vi "HAR-15-001-RecordingStimulation_BL.vi"() -> ()   [LabVIEW 2014]
doc: "I. Description:\nThis example demonstrates how to continuously acquire unscaled and save the data in a binary file. You can use the Graph Acquired Binary Data.VI to read and plot the scaled data on a Waveform Graph.\n\nII. Instructions for Running:\n1. Select the physical channel to correspond to where your signal is input on the DAQ device.\n2. Enter the minimum and maximum voltage ranges.\nNote: For better accuracy try to match the input range to the expected voltage level of the measured signal.\n3. Set the rate of the acquisition Also set the Samples to Read control. This will determine how many samples are read each time the while loop iterates. This also determines how many points are plotted on the graph each iteration.\nNote: The rate should be at least twice as fast as the maximum frequency component of the signal being acquired.\n4. Select the File Properties. If the file path is left empty, it will bring up a dialog box to let you browse to the file. \n\nIII. Block Diagram Steps:\n1. Create or replace a file to store the data.\n2. Create an analog input voltage channel.\n3. Set the rate for the sample clock. Additionally, define the sample mode to be continuous.\n4. Create a header and write it to the binary file.\n5. Call the Start VI to start acquiring samples. \n6. Read the unscaled data in a loop until the user hits the stop button or an error occurs.\nNote: This example uses unscaled I32 reads. Some devices support unscaled reads in smaller widths, such as I16. To get the maximum performance out of your device, use the unscaled read with the smallest supported width.\n7. Transpose the unscaled array of data and append it to the file.\n8. Close the File.\n9. Call the Stop VI to stop acquiring samples.\n10. Use the popup dialog box to display an error if any.\n\nIV. I/O Connections Overview:\nMake sure your signal input terminal matches the Physical Channel I/O control. For further connection information, refer to your hardware reference manual."
uses:
  <vilib>/Utility/error.llb/DialogType.ctl
  <vilib>/DAQmx/read.llb/DAQmx Read (Analog 2D I32 NChan NSamp).vi
  <vilib>/DAQmx/create/channels.llb/DAQmx Create Channel (AI-Voltage-Basic).vi
  <vilib>/DAQmx/configure/timing.llb/DAQmx Timing (Sample Clock).vi
  <vilib>/DAQmx/miscellaneous.llb/DAQmx Fill In Error Info.vi
  <vilib>/Utility/file.llb/Read From Spreadsheet File (string).vi
  <vilib>/Waveform/DWDTOps.llb/DWDT Boolean Array to Digital.vi
panel:
  out "AMP Thres":dbl
  in  "WinEnd":i32
  in  "WinStart":i32
  in  "Y Scale Range":dbl=10.0
  out "StimulationCounter":i32
  out "?":i32
  in  "?":u16(ring) items=["TC1", "TC2", "TC3", "TC4", "TC5", "TC6", "TC7", "TC8", "TC9", "TC10"]
  out "TC On?":bool
  in  "?":bool
  out "Orders":i32[][](array[numeric])
  out "StimulationSetting":T1(array[cluster])
  in  "?":enum32{"ES1", "ES 2", "TMS"}(radio)
  out "Files Opens":bool[](array[boolean])
  out "1st Event Position":dbl
  out "Group of ES set":i32
  out "File Writing Array":bool[](array[boolean])
  out "Single File RefNum":refnum<file>
  out "Files RefNum":refnum<file>[](array[refnum])
  out "Cursor Auto Jump":bool
  in  "Curor Auto Jump":bool=TRUE
  in  "?":bool
  out "STDP On?":bool
  out "# Events":u32
  out "# Reps Left":dbl
  in  "Tab Control":T2(tab)
  out "R APB":dbl[][](graph)
  out "R ADM":dbl[][](graph)
  out "R APB AMP":dbl
  out "R ADM AMP":dbl
  out "R APB +":i32
  out "R APB -":i32
  out "R ADM -":i32
  out "R ADM +":i32
  out "L ADM -":i32
  out "L ADM +":i32
  out "L APB -":i32
  out "L APB +":i32
  out "L ADM AMP":dbl
  out "L APB AMP":dbl
  out "L APB":dbl[][](graph)
  out "L ADM":dbl[][](graph)
  out "R BI":dbl[][](graph)
  out "R BI AMP":dbl
  out "R BI +":i32
  out "R BI -":i32
  out "L BI":dbl[][](graph)
  out "L BI -":i32
  out "L BI +":i32
  out "L BI AMP":dbl
  out "L FCR":dbl[][](graph)
  out "L FCR AMP":dbl
  out "L FCR +":i32
  out "L FCR -":i32
  out "R FCR":dbl[][](graph)
  out "R FCR -":i32
  out "R FCR +":i32
  out "R FCR AMP":dbl
  out "Looping Iteration":i16
  in  "Repetitions":i8=5
  in  "TMS Delay Interval":dbl max=250.0
  out "TMS Delay Interval (ms)":dbl(slide) scale=0.0..250.0
  in  "TMS Interval":dbl=40.0
  out "ES 2 Delay Interval (ms)":dbl(slide) scale=0.0..250.0
  in  "ES2 Delay Interval":dbl max=250.0
  in  "ES2 Interval":dbl=40.0
  in  "ES1 Delay Interval":dbl max=250.0
  out "ES 1 Delay Interval (ms)":dbl(slide) max=100.0 scale=0.0..250.0
  in  "ES1 Interval":dbl=40.0
  in  "Trigger Pulse Width (Points)":i16=5
  in  "Rate - every X s":dbl=5.0
  in  "?":bool
  in  "Looping Switch":bool
  in  "Buffered Size":i16=2500
  in  "Sampling Rate":dbl=10000.0
  out "ES1 On?":bool
  out "ES2 On?":bool
  out "TMS On?":bool
  in  "TMS Activate":bool=TRUE
  in  "ES1 Activate":bool=TRUE
  in  "ES2 Activate":bool=TRUE
  out "ES1 DP On?":bool
  out "ES2 DP On?":bool
  out "TMS Doublet On?":bool
  in  "ES1 Doublet On?":bool
  in  "ES2 Doublet On?":bool
  in  "TMS Doublet On?":bool
  out "peak X value":dbl
  out "Peak Count":i32
  in  "peak number":i32
  in  "Cursor Jump":bool
  out "S1":dbl[][](graph)
  in  "stop B":bool
  in  "stop A":bool
  in  "# updates/sec":dbl=4.0
  out "volts/bit":dbl
  out "Samples Per Channel Per Iteration":dbl
  out "Time (sec)":dbl
  out "# channels":dbl
  out "Samples to Read":i32=1
  in  "Maximum Value":dbl=10.0 format="%0.2f"
  in  "Minimum Value":dbl=-10.0 format="%0.2f"
  in  "DAQ Channels":tag="Dev3/ai0:7, Dev3/ai16:18" caption="Channel List"
  # "File Properties"
  # "Channel Parameters"
  # "Advanced Setting For DO"
  # "Timing Parameters"
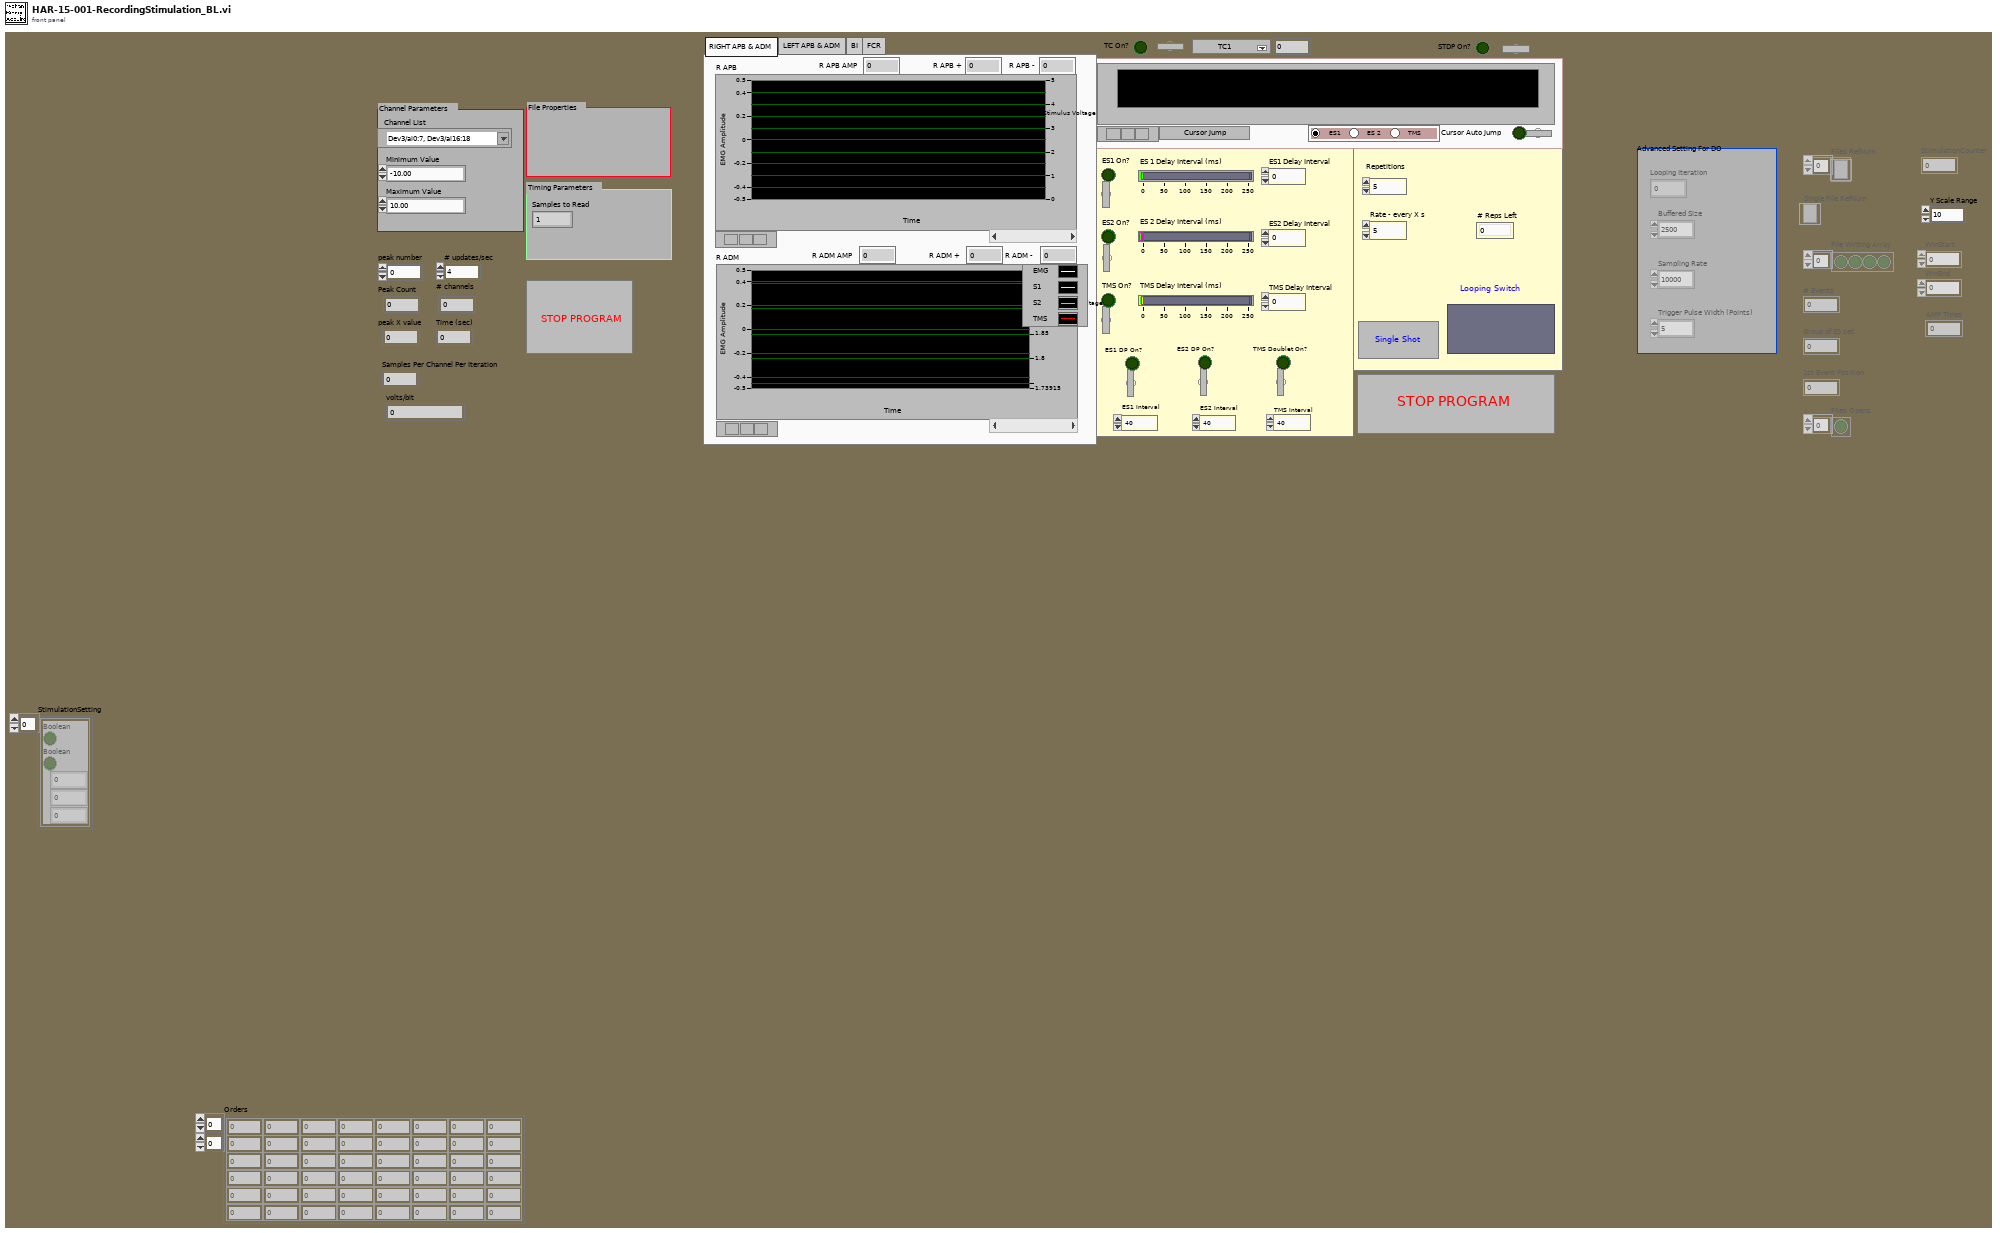
[diagram p1: front panel]
types:
  T1 = cluster{"Boolean":bool, "Boolean":bool, dbl, dbl, dbl}[]
  T2 = enum32{"RIGHT APB & ADM", "LEFT APB & ADM", "BI", "FCR"}
  T3 = typedef "DialogType.ctl" = u16
  T4 = cluster{"Boolean":bool, "Boolean":bool, dbl, dbl, dbl}
  T5 = enum16{"open", "open or create", "create or replace", "create", "open (read only)"}
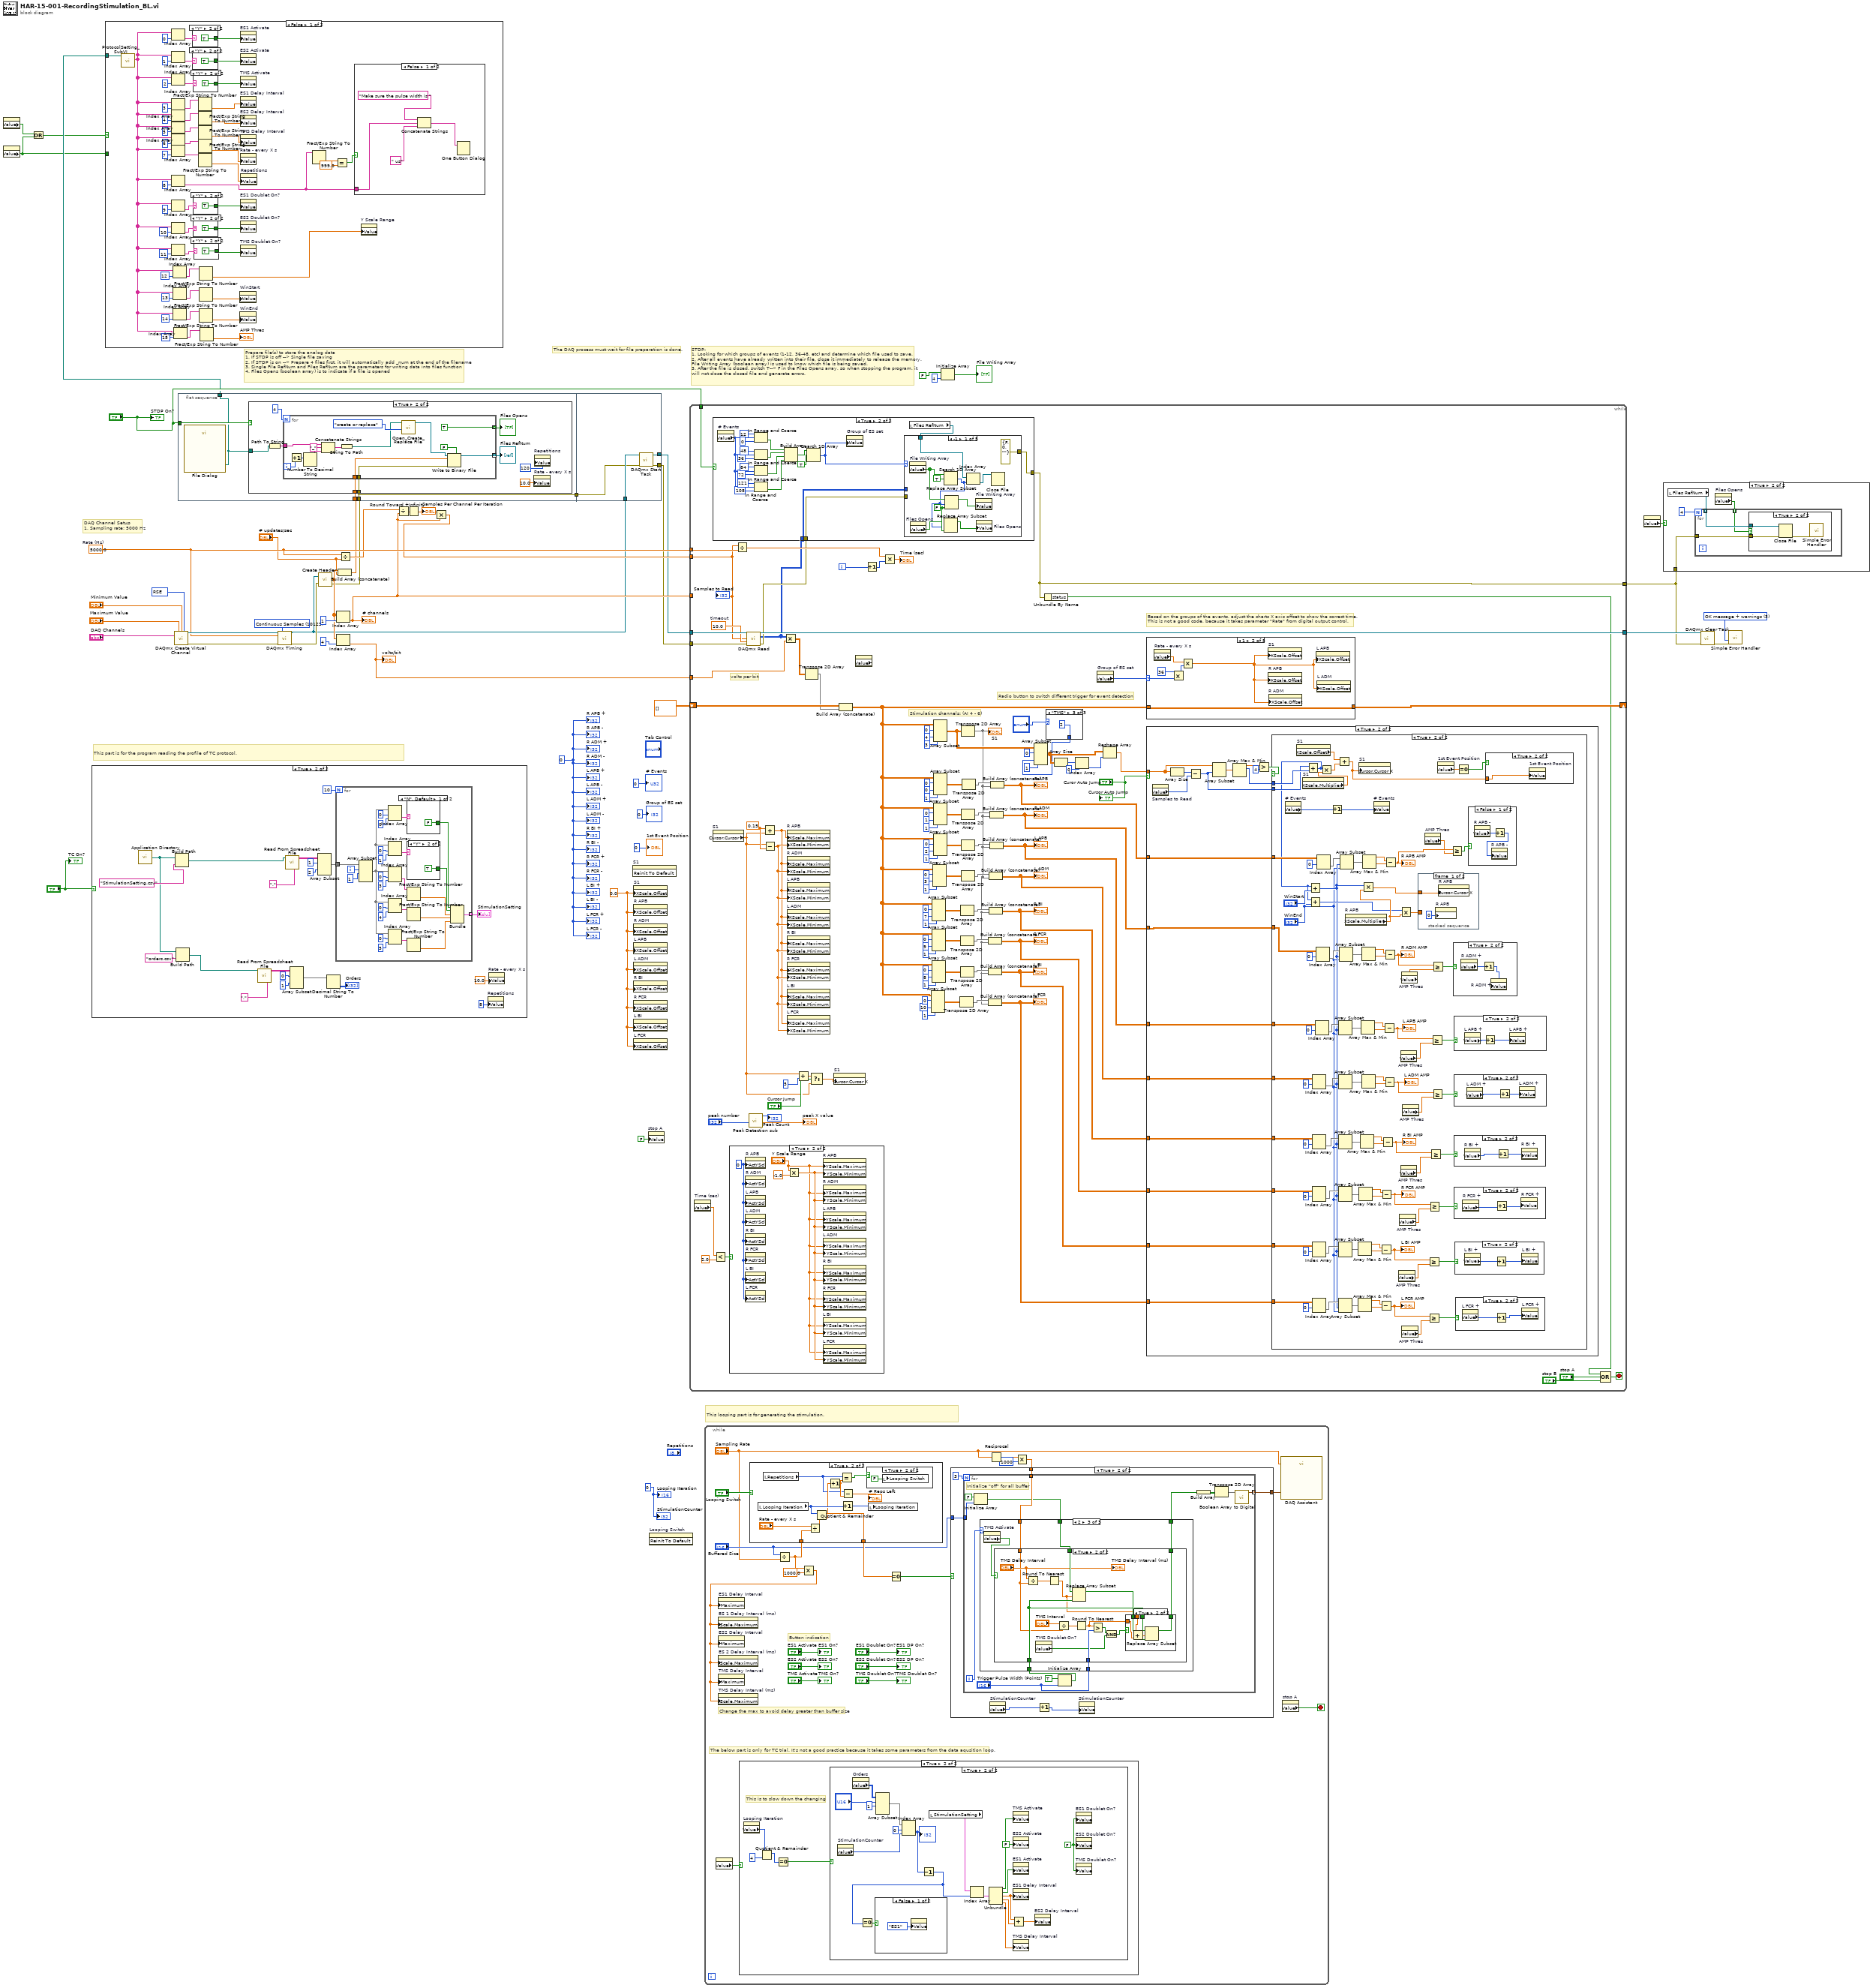
[diagram p0: block diagram]
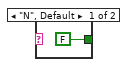
[diagram p3: hidden frame]
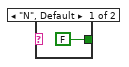
[diagram p4: hidden frame]
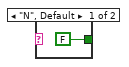
[diagram p5: hidden frame]
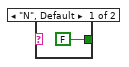
[diagram p6: hidden frame]
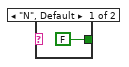
[diagram p7: hidden frame]
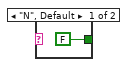
[diagram p8: hidden frame]
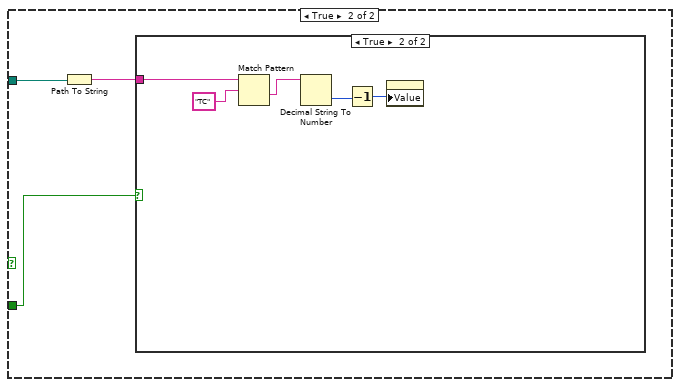
[diagram p9: hidden frame]
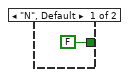
[diagram p12: hidden frame]
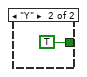
[diagram p13: hidden frame]
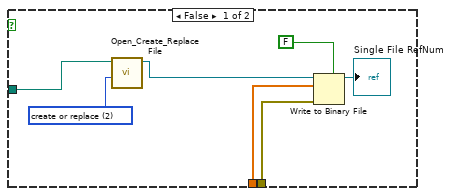
[diagram p14: hidden frame]
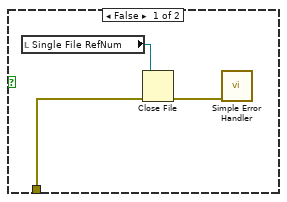
[diagram p15: hidden frame]
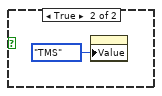
[diagram p19: hidden frame]
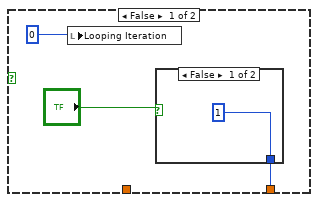
[diagram p20: hidden frame]
diagram:
  w2 = 0
  w1 = 0.0 ("X Scale.Offset and Multiplier:Offset")
  w10 = 0
  w35 = 5000.0  # Rate (Hz)
  w41 = 10083 items=["default"=-1, "RSE"=10083, "NRSE"=10078, "Differential"=10106, "Pseudodifferential"=12529] ("input terminal configuration")
  w43 = T3 3 items=["no dialog", "OK message", "continue or stop message", "OK message + warnings", "continue/stop + warnings"] ("type of dialog (OK msg:1)")
  w45 = 10123 items=["Finite Samples"=10178, "Continuous Samples"=10123] ("sample mode")
  # "This looping part is for generating the stimulation."
  # "This part is for the program reading the profile of TC protocol."
  # "STDP:\n1. Looking for which groups of events (1-12, 36-48, etc) and determine which file used to save.\n2. After all events have already written into their file, close it immediately to release the memory.\nFile Writing Array (boolean array) is used to know which file is being saved.\n3. After the file is closed, switch T--> F in the Files Opens array, so when stopping the program, it\nwill not close the closed file and generate errors."
  # "The DAQ process must wait for file preparation is done."
  # "DAQ Channel Setup\n1. Sampling rate: 5000 Hz"
  # "Prepare file(s) to store the analog data\n1. If STDP is off --> Single file saving\n2. If STDP is on --> Prepare 4 files first, it will automatically add _num at the end of the filename\n3. Single File RefNum and Files RefNum are the parameters for writing data into files function\n4. Files Opens (boolean array) is to indicate if a file is opened"
  n1 = property class="Bool (strict)"() -> ("Value"=w6:bool)  [unwired: 2 in, 2 out]
  n2 = property class="Bool (strict)"() -> ("Value"=w3:bool)  [unwired: 2 in, 2 out]
  n3 = Or(x=w6, y=w3) -> (x .or. y?=w5:bool)
  n4 = case shown="True" "?" {
    frame False {
    }
    frame True {
      n5 = call <vilib>:"Application Directory.vi"() -> ("Application Directory"=w50:path)
      n6 = Build Path(base path=w50, name or relative path="StimulationSetting.csv" ("file path (dialog if empty)")) -> (appended path=w51:path)
      n7 = Build Path(base path=w50, name or relative path="orders.csv") -> (appended path=w48:path)
      n8 = call-poly <vilib>:"Read From Spreadsheet File.vi"("delimiter (\\t)"="," ("delimiter (\\t)"), "file path (dialog if empty)"=w48) -> ("all rows"=w59:string[][])  [unwired: 5 in, 4 out]
      n9 = call-poly <vilib>:"Read From Spreadsheet File.vi"("delimiter (\\t)"="," ("delimiter (\\t)"), "file path (dialog if empty)"=w51) -> ("all rows"=w66:string[][])  [unwired: 5 in, 4 out]
      n10 = Array Subset(array=w59, index (row)=0 ("index"), index (col)=1 ("index")) -> (w56:string[][])  [unwired: 2 in]
      n11 = Array Subset(array=w66, index (row)=1 ("index"), index (col)=2 ("index")) -> (w63:string[][])  [unwired: 2 in]
      n12 = Decimal String To Number(string=w56) -> (number=→"Orders":i32[][])  [unwired: 2 in, 1 out]
      n13 = for {
        N: 10 -> [_]
        tunnel: w63 -> [w92]
        tunnel: [w68] -> w61 mode=indexing
        i -> [w74]
        n14 = Array Subset(array=w92, index (row)=w74, length (row)=1 ("length")) -> (w78:string[][])  [unwired: 2 in]
        n15 = Index Array(array=w78, index (row)=0, index (col)=0 ("disabled index (col)")) -> (element=w88:string)
        n16 = Index Array(array=w78, index (row)=0, index (col)=1 ("disabled index (col)")) -> (element=w85:string)
        n17 = Index Array(array=w78, index (row)=0, index (col)=3 ("disabled index (col)")) -> (element=w75:string)
        n18 = Index Array(array=w78, index (row)=0, index (col)=4 ("disabled index (col)")) -> (element=w76:string)
        n19 = Index Array(array=w78, index (row)=0, index (col)=5 ("disabled index (col)")) -> (element=w77:string)
        n20 = case shown="\"N\", Default" w88 {
          tunnel: [FALSE ("Boolean") TRUE ("Boolean")] -> w73
          frame "N", Default {
          }
          frame "Y" {
          }
        }
        n21 = case shown="\"Y\"" w85 {
          tunnel: [FALSE ("Boolean") TRUE ("Boolean")] -> w72
          frame "N", Default {
          }
          frame "Y" {
          }
        }
        n22 = Fract/Exp String To Number(string=w75) -> (number=w71:dbl)  [unwired: 3 in, 1 out]
        n23 = Fract/Exp String To Number(string=w76) -> (number=w70:dbl)  [unwired: 3 in, 1 out]
        n24 = Fract/Exp String To Number(string=w77) -> (number=w69:dbl)  [unwired: 3 in, 1 out]
        n25 = Bundle("Boolean"=w73, "Boolean"=w72, w71, w70, w69) -> (w68:T4)  [unwired: 1 in]
      }
      "StimulationSetting" <- w61
      n26 = property on="Repetitions" class="DigNum (strict)"("Value"=i8 8 ("Repetitions")) -> ()  [unwired: 2 in, 2 out]
      n27 = property on="Rate - every X s" class="DigNum (strict)"("Value"=10.0 ("Rate - every X s")) -> ()  [unwired: 2 in, 2 out]
    }
  }
  n28 = case shown="False" w5 {
    tunnel: w9 -> [w117 w166]
    tunnel: w3 -> [_ w165]
    frame False {
      n29 = call "ProtocolSetting_SubVI.vi"("selected path"=w117) -> ("all rows"=w99:string[])  [unwired: 9 in, 1 out]
      n30 = Index Array(array=w99, index=0) -> (element=w147:string)
      n31 = Index Array(array=w99, index=1) -> (element=w144:string)
      n32 = Index Array(array=w99, index=2) -> (element=w142:string)
      n33 = Index Array(array=w99, index=3) -> (element=w139:string)
      n34 = Index Array(array=w99, index=4) -> (element=w138:string)
      n35 = Index Array(array=w99, index=5) -> (element=w137:string)
      n36 = Index Array(array=w99, index=6) -> (element=w136:string)
      n37 = Index Array(array=w99, index=7) -> (element=w132:string)
      n38 = Index Array(array=w99, index=8) -> (element=w110:string)
      n39 = Index Array(array=w99, index=9) -> (element=w131:string)
      n40 = Index Array(array=w99, index=10) -> (element=w130:string)
      n41 = Index Array(array=w99, index=11) -> (element=w129:string)
      n42 = Index Array(array=w99, index=12) -> (element=w108:string)
      n43 = Index Array(array=w99, index=13) -> (element=w104:string)
      n44 = Index Array(array=w99, index=14) -> (element=w103:string)
      n45 = Index Array(array=w99, index=15) -> (element=w98:string)
      n46 = case shown="\"Y\"" w147 {
        tunnel: [FALSE TRUE] -> w146
        frame "N", Default {
        }
        frame "Y" {
        }
      }
      n47 = case shown="\"Y\"" w144 {
        tunnel: [FALSE TRUE] -> w141
        frame "N", Default {
        }
        frame "Y" {
        }
      }
      n48 = case shown="\"Y\"" w142 {
        tunnel: [FALSE TRUE] -> w140
        frame "N", Default {
        }
        frame "Y" {
        }
      }
      n49 = case shown="\"Y\"" w131 {
        tunnel: [FALSE TRUE] -> w120
        frame "N", Default {
        }
        frame "Y" {
        }
      }
      n50 = case shown="\"Y\"" w130 {
        tunnel: [FALSE TRUE] -> w119
        frame "N", Default {
        }
        frame "Y" {
        }
      }
      n51 = case shown="\"Y\"" w129 {
        tunnel: [FALSE TRUE] -> w118
        frame "N", Default {
        }
        frame "Y" {
        }
      }
      n52 = Fract/Exp String To Number(string=w139) -> (number=w135:dbl)  [unwired: 3 in, 1 out]
      n53 = Fract/Exp String To Number(string=w138) -> (number=w134:dbl)  [unwired: 3 in, 1 out]
      n54 = Fract/Exp String To Number(string=w137) -> (number=w133:dbl)  [unwired: 3 in, 1 out]
      n55 = Fract/Exp String To Number(string=w136) -> (number=w115:dbl)  [unwired: 3 in, 1 out]
      n56 = Fract/Exp String To Number(string=w132) -> (number=w114:dbl)  [unwired: 3 in, 1 out]
      n57 = Fract/Exp String To Number(string=w108) -> (number=w107:dbl)  [unwired: 3 in, 1 out]
      n58 = Fract/Exp String To Number(string=w104) -> (number=w102:dbl)  [unwired: 3 in, 1 out]
      n59 = Fract/Exp String To Number(string=w103) -> (number=w101:dbl)  [unwired: 3 in, 1 out]
      n60 = Fract/Exp String To Number(string=w98) -> (number=→"AMP Thres":dbl)  [unwired: 3 in, 1 out]
      n61 = property on="WinStart" class="DigNum (strict)"("Value"=w102) -> ()  [unwired: 2 in, 2 out]
      n62 = property on="WinEnd" class="DigNum (strict)"("Value"=w101) -> ()  [unwired: 2 in, 2 out]
      n63 = property on="ES1 Activate" class="Bool (strict)"("Value"=w146) -> ()  [unwired: 2 in, 2 out]
      n64 = property on="ES2 Activate" class="Bool (strict)"("Value"=w141) -> ()  [unwired: 2 in, 2 out]
      n65 = property on="TMS Activate" class="Bool (strict)"("Value"=w140) -> ()  [unwired: 2 in, 2 out]
      n66 = property on="ES1 Delay Interval" class="DigNum (strict)"("Value"=w135) -> ()  [unwired: 2 in, 2 out]
      n67 = property on="ES2 Delay Interval" class="DigNum (strict)"("Value"=w134) -> ()  [unwired: 2 in, 2 out]
      n68 = property on="TMS Delay Interval" class="DigNum (strict)"("Value"=w133) -> ()  [unwired: 2 in, 2 out]
      n69 = property on="Rate - every X s" class="DigNum (strict)"("Value"=w115) -> ()  [unwired: 2 in, 2 out]
      n70 = property on="ES1 Doublet On?" class="Bool (strict)"("Value"=w120) -> ()  [unwired: 2 in, 2 out]
      n71 = property on="ES2 Doublet On?" class="Bool (strict)"("Value"=w119) -> ()  [unwired: 2 in, 2 out]
      n72 = property on="TMS Doublet On?" class="Bool (strict)"("Value"=w118) -> ()  [unwired: 2 in, 2 out]
      n73 = property on="Repetitions" class="DigNum (strict)"("Value"=w114) -> ()  [unwired: 2 in, 2 out]
      n74 = Fract/Exp String To Number(string=w110) -> (number=w113:dbl)  [unwired: 3 in, 1 out]
      n75 = Equal?(x=w113, y=999.0) -> (x = y?=w111:bool)
      n76 = case shown="False" w111 {
        tunnel: w110 -> [w152 _]
        frame False {
          n77 = Concatenate Strings("Make sure the pulse width is ", w152, " us" ("string")) -> (w149:string)
          n78 = One Button Dialog(message=w149) -> ()  [unwired: 1 in, 1 out]
        }
        frame True {
        }
      }
      n79 = property on="Y Scale Range" class="DigNum (strict)"("Value"=w107) -> ()  [unwired: 2 in, 2 out]
    }
    frame True {
      n80 = Path To String(path=w166) -> (string=w167:string)
      n81 = case shown="True" w165 {
        tunnel: w167 -> [_ w172]
        frame False {
        }
        frame True {
          n82 = Match Pattern(string=w172, regular expression="TC") -> (after substring=w170:string)  [unwired: 1 in, 3 out]
          n83 = Decimal String To Number(string=w170) -> (number=w169:i32)  [unwired: 2 in, 1 out]
          n84 = Decrement(x=w169) -> (x-1=w168:i32)
          n85 = property class="Ring (strict)"("Value"=w168) -> ()  [unwired: 2 in, 2 out]
        }
      }
    }
  }
  n86 = call-poly <vilib>:"DAQmx Create Virtual Channel.vi"("maximum value"="Maximum Value", "minimum value"="Minimum Value", "input terminal configuration"=w41, "physical channels"="DAQ Channels") -> ("task out"=w40:refnum<k21>, "error out"=w39:errorcluster)  [unwired: 5 in, 5 out]
  n87 = flat-sequence {
    tunnel: [w176] -> w8
    tunnel: [w173] -> w9
    tunnel: w21 -> [w176]
    tunnel: w23 -> [w174]
    tunnel: "?" -> [w175]
    tunnel: [w210] -> w20
    tunnel: [w209] -> w19
    tunnel: w7 -> [w208]
    tunnel: w8 -> [w207]
    frame #0 {
      n88 = call "File Dialog"() -> ("selected path"=w173:path)  [unwired: 12 in, 3 out]
      n89 = case shown="True" w175 {
        tunnel: w174 -> [w183 w190]
        tunnel: w176 -> [w180 w189]
        tunnel: w173 -> [w177 w186]
        frame False {
          w179 = i16 2 items=["open", "open or create", "create or replace", "create"] ("function")
          n90 = call <vilib>:"Open_Create_Replace File.vi"("function (open:0)"=w179, "file path"=w177) -> ("refnum"=w178:refnum<file>)  [unwired: 4 in, 5 out]
          n91 = Write to Binary File(file (use dialog)=w178, data=w183, error in=w180, 5:FALSE ("prepend array or string size? (T)")) -> (refnum out=→"Single File RefNum":refnum<file>)  [unwired: 4 out]
        }
        frame True {
          n92 = Path To String(path=w186) -> (string=w192:string)
          n93 = for {
            N: 4 -> [_]
            tunnel: w192 -> [w206]
            tunnel: [w196] -> w188 mode=indexing
            tunnel: w190 -> [w195]
            tunnel: w189 -> [w194]
            tunnel: [TRUE] -> w187 mode=indexing
            i -> [w205]
            n94 = Increment(x=w205) -> (x+1=w204:i32)
            n95 = Number To Decimal String(number=w204) -> (decimal integer string=w203:string)  [unwired: 1 in]
            n96 = Concatenate Strings(w206, "_" ("string"), w203) -> (w200:string)
            n97 = String To Path(string=w200) -> (path=w198:path)
            n98 = call <vilib>:"Open_Create_Replace File.vi"("function (open:0)"=T5."create or replace", "file path"=w198) -> ("refnum"=w197:refnum<file>)  [unwired: 4 in, 5 out]
            n99 = Write to Binary File(file (use dialog)=w197, data=w195, error in=w194, 5:FALSE ("prepend array or string size? (T)")) -> (refnum out=w196:refnum<file>)  [unwired: 4 out]
          }
          "Files RefNum" <- w188
          "Files Opens" <- w187
          n100 = property on="Rate - every X s" class="DigNum (strict)"("Value"=10.0 ("Rate - every X s")) -> ()  [unwired: 2 in, 2 out]
          n101 = property on="Repetitions" class="DigNum (strict)"("Value"=i8 120 ("Repetitions")) -> ()  [unwired: 2 in, 2 out]
        }
      }
    }
    frame #1 {
      n102 = call <vilib>:"DAQmx Start Task.vi"("task/channels in"=w208, "error in"=w207) -> ("task out"=w210:refnum<k21>, "error out"=w209:errorcluster)  [unwired: 12 out]
    }
  }
  n103 = call-poly <vilib>:"DAQmx Timing.vi"("task/channels in"=w40, "sample mode"=w45, "rate"=w35, "error in"=w39) -> ("task out"=w7:refnum<k21>, "error out"=w44:errorcluster)  [unwired: 3 in, 7 out]
  n104 = call "Create Header.vi"("task in"=w7, "error in"=w44) -> ("Array"=w27:dbl[], "error out"=w21:errorcluster)  [unwired: 1 out]
  n105 = Index Array(array=w27, index=1) -> (element=w31:dbl)
  "# channels" <- w31
  n106 = Index Array(array=w27, index=4) -> (element=w28:dbl)
  "volts/bit" <- w28
  n107 = Build Array (concatenate)(w27, "# updates/sec") -> (w23:dbl[])
  n108 = Divide(x=w35, y="# updates/sec") -> (x/y=w34:dbl)
  n109 = Divide(x=w34, y=w31) -> (x/y=w33:dbl)
  n110 = Round Toward +Infinity(x=w33) -> (ceil(x): smallest int >= x=w32:dbl)
  "Samples Per Channel Per Iteration" <- w32
  n111 = Multiply(x=w32, y=w31) -> (x*y=w30:dbl)
  n112 = invoke on="S1" class="WFGraph (strict)" method="Reinit To Default"() -> ()  [unwired: 3 in, 3 out]
  n113 = property on="S1" class="WFGraph (strict)"("XScale.Offset"=w1) -> ()  [unwired: 2 in, 2 out]
  n114 = property on="R APB" class="WFGraph (strict)"("XScale.Offset"=w1) -> ()  [unwired: 2 in, 2 out]
  n115 = property on="R ADM" class="WFGraph (strict)"("XScale.Offset"=w1) -> ()  [unwired: 2 in, 2 out]
  n116 = property on="L APB" class="WFGraph (strict)"("XScale.Offset"=w1) -> ()  [unwired: 2 in, 2 out]
  n117 = property on="L ADM" class="WFGraph (strict)"("XScale.Offset"=w1) -> ()  [unwired: 2 in, 2 out]
  n118 = property on="R BI" class="WFGraph (strict)"("XScale.Offset"=w1) -> ()  [unwired: 2 in, 2 out]
  n119 = property on="R FCR" class="WFGraph (strict)"("XScale.Offset"=w1) -> ()  [unwired: 2 in, 2 out]
  n120 = property on="L BI" class="WFGraph (strict)"("XScale.Offset"=w1) -> ()  [unwired: 2 in, 2 out]
  n121 = property on="L FCR" class="WFGraph (strict)"("XScale.Offset"=w1) -> ()  [unwired: 2 in, 2 out]
  n122 = property on="stop A" class="Bool (strict)"("Value"=FALSE ("stop A")) -> ()  [unwired: 2 in, 2 out]
  n123 = invoke on="Looping Switch" class="Bool (strict)" method="Reinit To Default"() -> ()  [unwired: 3 in, 3 out]
  n124 = while {
    tunnel: w19 -> [w312]
    tunnel: w20 -> [w311]
    tunnel: [w310] -> w47
    tunnel: [w295] -> w13
    tunnel: w31 -> [_]
    tunnel: w28 -> [w297]
    tunnel: w35 -> [w308]
    tunnel: w30 -> [w307]
    tunnel: "?" -> [w299]
    shift-right: [w250] -> _
    shift-left: dbl[][] [] -> [w298]
    i -> [w306]
    stop <- w244 stop-if-true
    w293 = 0.15
    w309 = 10.0  # timeout
    # "Based on the groups of the events, adjust the charts X axis offset to show the correct time.\nThis is not a good code, because it takes parameter \"Rate\" from digital output control."
    # "Radio button to switch different trigger for event detection"
    # "Stimulation channels: (AI 4 - 6)"
    # "volts per bit"
    n125 = property on="Time (sec)" class="DigNum (strict)"() -> ("Value"=w212:dbl)  [unwired: 2 in, 2 out]
    n126 = property on="S1" class="WFGraph (strict)"() -> ("Cursor.Cursor X"=w288:dbl)  [unwired: 2 in, 2 out]
    n127 = Less?(x=w212, y=2.0) -> (x < y?=w213:bool)
    n128 = case shown="True" w213 {
      frame False {
      }
      frame True {
        w315 = 0 ("Active Y Scale")
        n129 = property on="R APB" class="WFGraph (strict)"("ActYScl"=w315) -> ()  [unwired: 2 in, 2 out]
        n130 = property on="R ADM" class="WFGraph (strict)"("ActYScl"=w315) -> ()  [unwired: 2 in, 2 out]
        n131 = property on="L APB" class="WFGraph (strict)"("ActYScl"=w315) -> ()  [unwired: 2 in, 2 out]
        n132 = property on="L ADM" class="WFGraph (strict)"("ActYScl"=w315) -> ()  [unwired: 2 in, 2 out]
        n133 = property on="R BI" class="WFGraph (strict)"("ActYScl"=w315) -> ()  [unwired: 2 in, 2 out]
        n134 = property on="R FCR" class="WFGraph (strict)"("ActYScl"=w315) -> ()  [unwired: 2 in, 2 out]
        n135 = property on="L BI" class="WFGraph (strict)"("ActYScl"=w315) -> ()  [unwired: 2 in, 2 out]
        n136 = property on="L FCR" class="WFGraph (strict)"("ActYScl"=w315) -> ()  [unwired: 2 in, 2 out]
        n137 = Multiply(x="Y Scale Range", y=-1.0) -> (x*y=w314:dbl)
        n138 = property on="R APB" class="WFGraph (strict)"("YScale.Maximum"="Y Scale Range", "YScale.Minimum"=w314) -> ()  [unwired: 2 in, 2 out]
        n139 = property on="R ADM" class="WFGraph (strict)"("YScale.Maximum"="Y Scale Range", "YScale.Minimum"=w314) -> ()  [unwired: 2 in, 2 out]
        n140 = property on="L APB" class="WFGraph (strict)"("YScale.Maximum"="Y Scale Range", "YScale.Minimum"=w314) -> ()  [unwired: 2 in, 2 out]
        n141 = property on="L ADM" class="WFGraph (strict)"("YScale.Maximum"="Y Scale Range", "YScale.Minimum"=w314) -> ()  [unwired: 2 in, 2 out]
        n142 = property on="R BI" class="WFGraph (strict)"("YScale.Maximum"="Y Scale Range", "YScale.Minimum"=w314) -> ()  [unwired: 2 in, 2 out]
        n143 = property on="R FCR" class="WFGraph (strict)"("YScale.Maximum"="Y Scale Range", "YScale.Minimum"=w314) -> ()  [unwired: 2 in, 2 out]
        n144 = property on="L BI" class="WFGraph (strict)"("YScale.Maximum"="Y Scale Range", "YScale.Minimum"=w314) -> ()  [unwired: 2 in, 2 out]
        n145 = property on="L FCR" class="WFGraph (strict)"("YScale.Maximum"="Y Scale Range", "YScale.Minimum"=w314) -> ()  [unwired: 2 in, 2 out]
      }
    }
    n146 = Divide(x=w307, y=w308) -> (x/y=w303:dbl)
    n147 = call-poly <vilib>:"DAQmx Read.vi"("task/channels in"=w311, "number of samples per channel"=w307, "timeout"=w309, "error in"=w312) -> ("task out"=w310:refnum<k21>, "data"=w294:i32[][], "error out"=w300:errorcluster)  [unwired: 9 out]
    n148 = case shown="True" w299 {
      tunnel: w294 -> [w488 w493]
      tunnel: w300 -> [w486 w492]
      tunnel: [w484 w491] -> w295
      frame False {
        n149 = local read "Single File RefNum"() -> (w485:refnum<file>)
        n150 = Write to Binary File(file (use dialog)=w485, data=w488, error in=w486, 5:FALSE ("prepend array or string size? (T)")) -> (error out=w484:errorcluster)  [unwired: 4 out]
      }
      frame True {
        n151 = property on="# Events" class="DigNum (strict)"() -> ("Value"=w500:u32)  [unwired: 2 in, 2 out]
        n152 = In Range and Coerce(upper limit=u32 12, x=w500, lower limit=u32 0) -> (In Range?=w499:bool)  [unwired: 1 out]
        n153 = In Range and Coerce(upper limit=u32 48, x=w500, lower limit=u32 36) -> (In Range?=w498:bool)  [unwired: 1 out]
        n154 = In Range and Coerce(upper limit=u32 84, x=w500, lower limit=u32 72) -> (In Range?=w497:bool)  [unwired: 1 out]
        n155 = In Range and Coerce(upper limit=u32 121, x=w500, lower limit=u32 108) -> (In Range?=w496:bool)  [unwired: 1 out]
        n156 = Build Array(w499, w498, w497, w496) -> (w495:bool[])
        n157 = Search 1D Array(1D array=w495, element=TRUE) -> (index of element=w489:i32)  [unwired: 1 in]
        n158 = property on="Group of ES set" class="DigNum (strict)"("Value"=w489) -> ()  [unwired: 2 in, 2 out]
        n159 = local read "Files RefNum"() -> (w490:refnum<file>[])
        n160 = case shown="-1" w489 {
          selector: w489 -> [_ w521 w531 w541 w551]
          tunnel: w490 -> [w516 w524 w534 w544 w554]
          tunnel: w493 -> [_ w527 w537 w547 w557]
          tunnel: w492 -> [_ w526 w536 w546 w556]
          tunnel: [errorcluster {"status"=FALSE, "code"=0, "source"=""} ("error out") w525 w535 w545 w555] -> w491
          frame -1 {
            w512 = FALSE ("new element/subarray")
            n161 = property on="File Writing Array" class="Arr (strict)"() -> ("Value"=w515:bool[])  [unwired: 2 in, 2 out]
            n162 = property on="Files Opens" class="Arr (strict)"() -> ("Value"=w511:bool[])  [unwired: 2 in, 2 out]
            n163 = Search 1D Array(1D array=w515, element=TRUE) -> (index of element=w510:i32)  [unwired: 1 in]
            n164 = Replace Array Subset(array=w511, new element=w512, index=w510) -> (w509:bool[])
            n165 = Replace Array Subset(array=w515, new element=w512, index=w510) -> (w514:bool[])
            n166 = Index Array(array=w516, index=w510) -> (element=w513:refnum<file>)
            n167 = property on="File Writing Array" class="Arr (strict)"("Value"=w514) -> ()  [unwired: 2 in, 2 out]
            n168 = property on="Files Opens" class="Arr (strict)"("Value"=w509) -> ()  [unwired: 2 in, 2 out]
            n169 = Close File(refnum=w513) -> ()  [unwired: 1 in, 2 out]
          }
          frame 0, Default {
            n170 = property on="File Writing Array" class="Arr (strict)"() -> ("Value"=w522:bool[])  [unwired: 2 in, 2 out]
            n171 = Index Array(array=w524, index=w521) -> (element=w523:refnum<file>)
            n172 = Replace Array Subset(array=w522, new element=TRUE ("new element/subarray"), index=w521) -> (w519:bool[])
            n173 = property on="File Writing Array" class="Arr (strict)"("Value"=w519) -> ()  [unwired: 2 in, 2 out]
            n174 = Write to Binary File(file (use dialog)=w523, data=w527, error in=w526, 5:FALSE ("prepend array or string size? (T)")) -> (error out=w525:errorcluster)  [unwired: 4 out]
          }
          frame 1 {
            n175 = property on="File Writing Array" class="Arr (strict)"() -> ("Value"=w532:bool[])  [unwired: 2 in, 2 out]
            n176 = Index Array(array=w534, index=w531) -> (element=w533:refnum<file>)
            n177 = Replace Array Subset(array=w532, new element=TRUE ("new element/subarray"), index=w531) -> (w529:bool[])
            n178 = property on="File Writing Array" class="Arr (strict)"("Value"=w529) -> ()  [unwired: 2 in, 2 out]
            n179 = Write to Binary File(file (use dialog)=w533, data=w537, error in=w536, 5:FALSE ("prepend array or string size? (T)")) -> (error out=w535:errorcluster)  [unwired: 4 out]
          }
          frame 2 {
            n180 = property on="File Writing Array" class="Arr (strict)"() -> ("Value"=w542:bool[])  [unwired: 2 in, 2 out]
            n181 = Index Array(array=w544, index=w541) -> (element=w543:refnum<file>)
            n182 = Replace Array Subset(array=w542, new element=TRUE ("new element/subarray"), index=w541) -> (w539:bool[])
            n183 = property on="File Writing Array" class="Arr (strict)"("Value"=w539) -> ()  [unwired: 2 in, 2 out]
            n184 = Write to Binary File(file (use dialog)=w543, data=w547, error in=w546, 5:FALSE ("prepend array or string size? (T)")) -> (error out=w545:errorcluster)  [unwired: 4 out]
          }
          frame 3 {
            n185 = property on="File Writing Array" class="Arr (strict)"() -> ("Value"=w552:bool[])  [unwired: 2 in, 2 out]
            n186 = Index Array(array=w554, index=w551) -> (element=w553:refnum<file>)
            n187 = Replace Array Subset(array=w552, new element=TRUE ("new element/subarray"), index=w551) -> (w549:bool[])
            n188 = property on="File Writing Array" class="Arr (strict)"("Value"=w549) -> ()  [unwired: 2 in, 2 out]
            n189 = Write to Binary File(file (use dialog)=w553, data=w557, error in=w556, 5:FALSE ("prepend array or string size? (T)")) -> (error out=w555:errorcluster)  [unwired: 4 out]
          }
        }
      }
    }
    n190 = call "Peak Detection sub.vi"("peak number"="peak number") -> ("x value of peak"=→"peak X value":dbl, "Count of Peaks"=→"Peak Count":i32)  [unwired: 9 in]
    n191 = Add(x=w293, y=w288) -> (x+y=w214:dbl)
    n192 = Subtract(x=w288, y=w293) -> (x-y=w215:dbl)
    n193 = Multiply(x=w294, y=w297) -> (x*y=w296:dbl[][])
    n194 = property on="R APB" class="WFGraph (strict)"("XScale.Maximum"=w214, "XScale.Minimum"=w215) -> ()  [unwired: 2 in, 2 out]
    n195 = property on="R ADM" class="WFGraph (strict)"("XScale.Maximum"=w214, "XScale.Minimum"=w215) -> ()  [unwired: 2 in, 2 out]
    n196 = property on="L APB" class="WFGraph (strict)"("XScale.Maximum"=w214, "XScale.Minimum"=w215) -> ()  [unwired: 2 in, 2 out]
    n197 = property on="L ADM" class="WFGraph (strict)"("XScale.Maximum"=w214, "XScale.Minimum"=w215) -> ()  [unwired: 2 in, 2 out]
    n198 = property on="R BI" class="WFGraph (strict)"("XScale.Maximum"=w214, "XScale.Minimum"=w215) -> ()  [unwired: 2 in, 2 out]
    n199 = property on="R FCR" class="WFGraph (strict)"("XScale.Maximum"=w214, "XScale.Minimum"=w215) -> ()  [unwired: 2 in, 2 out]
    n200 = property on="L BI" class="WFGraph (strict)"("XScale.Maximum"=w214, "XScale.Minimum"=w215) -> ()  [unwired: 2 in, 2 out]
    n201 = property on="L FCR" class="WFGraph (strict)"("XScale.Maximum"=w214, "XScale.Minimum"=w215) -> ()  [unwired: 2 in, 2 out]
    n202 = Add(x=w288, y=5) -> (x+y=w289:dbl)
    n203 = Transpose 2D Array(2D array=w296) -> (transposed array=w281:dbl[][])
    n204 = Select(t=w289, s="Cursor Jump", f=w288) -> (s? t:f=w292:dbl)
    n205 = property on="S1" class="WFGraph (strict)"("Cursor.Cursor X"=w292) -> ()  [unwired: 2 in, 2 out]
    n206 = Build Array (concatenate)(w298, w281) -> (w221:dbl[][])
    n207 = property class="Bool (strict)" props=["Value"]() -> ()  [unwired: 2 in, 3 out]
    n208 = Increment(x=w306) -> (x+1=w305:i32)
    n209 = Multiply(x=w303, y=w305) -> (x*y=→"Time (sec)":dbl)
    n210 = Array Subset(array=w221, index (row)=0 ("index"), index (col)=10 ("index"), length (col)=1 ("length")) -> (w223:dbl[][])  [unwired: 1 in]
    n211 = Array Subset(array=w221, index (row)=0 ("index"), index (col)=9 ("index"), length (col)=1 ("length")) -> (w233:dbl[][])  [unwired: 1 in]
    n212 = Array Subset(array=w221, index (row)=0 ("index"), index (col)=8 ("index"), length (col)=1 ("length")) -> (w228:dbl[][])  [unwired: 1 in]
    n213 = Array Subset(array=w221, index (row)=0 ("index"), index (col)=7 ("index"), length (col)=1 ("length")) -> (w238:dbl[][])  [unwired: 1 in]
    n214 = Array Subset(array=w221, index (row)=0 ("index"), index (col)=3 ("index"), length (col)=1 ("length")) -> (w262:dbl[][])  [unwired: 1 in]
    n215 = Array Subset(array=w221, index (row)=0 ("index"), index (col)=1 ("index"), length (col)=1 ("length")) -> (w272:dbl[][])  [unwired: 1 in]
    n216 = Array Subset(array=w221, index (row)=0 ("index"), index (col)=2 ("index"), length (col)=1 ("length")) -> (w267:dbl[][])  [unwired: 1 in]
    n217 = Array Subset(array=w221, index (row)=0 ("index"), index (col)=4 ("index"), length (col)=3 ("length")) -> (w259:dbl[][])  [unwired: 1 in]
    n218 = Array Subset(array=w221, index (row)=0 ("index"), index (col)=0 ("index"), length (col)=1 ("length")) -> (w277:dbl[][])  [unwired: 1 in]
    n219 = Transpose 2D Array(2D array=w223) -> (transposed array=w222:dbl[][])
    n220 = Transpose 2D Array(2D array=w233) -> (transposed array=w232:dbl[][])
    n221 = Transpose 2D Array(2D array=w228) -> (transposed array=w227:dbl[][])
    n222 = Transpose 2D Array(2D array=w238) -> (transposed array=w237:dbl[][])
    n223 = Transpose 2D Array(2D array=w262) -> (transposed array=w261:dbl[][])
    n224 = Transpose 2D Array(2D array=w259) -> (transposed array=w220:dbl[][])
    "S1" <- w220
    n225 = Transpose 2D Array(2D array=w272) -> (transposed array=w271:dbl[][])
    n226 = Transpose 2D Array(2D array=w267) -> (transposed array=w266:dbl[][])
    n227 = Transpose 2D Array(2D array=w277) -> (transposed array=w276:dbl[][])
    n228 = Build Array (concatenate)(w222, w220) -> (w216:dbl[][])
    "L FCR" <- w216
    n229 = Build Array (concatenate)(w232, w220) -> (w218:dbl[][])
    "R FCR" <- w218
    n230 = Build Array (concatenate)(w227, w220) -> (w217:dbl[][])
    "L BI" <- w217
    n231 = Build Array (concatenate)(w237, w220) -> (w219:dbl[][])
    "R BI" <- w219
    n232 = Build Array (concatenate)(w261, w220) -> (w242:dbl[][])
    "L ADM" <- w242
    n233 = Build Array (concatenate)(w271, w220) -> (w246:dbl[][])
    "R ADM" <- w246
    n234 = Build Array (concatenate)(w266, w220) -> (w243:dbl[][])
    "L APB" <- w243
    n235 = Build Array (concatenate)(w276, w220) -> (w247:dbl[][])
    "R APB" <- w247
    n236 = Unbundle By Name(w295) -> ("status"=w245:bool)
    n237 = case shown="\"TMS\"" "?" {
      tunnel: [0 1 2] -> w248
      frame "ES1", Default {
      }
      frame "ES 2" {
      }
      frame "TMS" {
      }
    }
    n238 = Array Subset(array=w259, index (row)=0 ("index"), index (col)=w248, length (col)=1 ("length")) -> (w255:dbl[][])  [unwired: 1 in]
    n239 = Array Size(array=w255) -> (size(s)=w254:i32[])
    n240 = Index Array(array=w254, index=0) -> (element=w252:i32)
    n241 = property on="Group of ES set" class="DigNum (strict)"() -> ("Value"=w251:i32)  [unwired: 2 in, 2 out]
    n242 = Reshape Array(w255, w252) -> (w256:dbl[])
    n243 = case shown="True" "Curor Auto Jump" {
      tunnel: w256 -> [_ w351]
      tunnel: w247 -> [_ w348]
      tunnel: w246 -> [_ w346]
      tunnel: w243 -> [_ w345]
      tunnel: w242 -> [_ w344]
      tunnel: w219 -> [_ w343]
      tunnel: w218 -> [_ w342]
      tunnel: w217 -> [_ w341]
      tunnel: w216 -> [_ w340]
      frame False {
      }
      frame True {
        n244 = property on="Samples to Read" class="DigNum (strict)"() -> ("Value"=w350:i32)  [unwired: 2 in, 2 out]
        n245 = Array Size(array=w351) -> (size(s)=w356:i32)
        n246 = Subtract(x=w356, y=w350) -> (x-y=w352:i32)
        n247 = Array Subset(array=w351, index=w352) -> (w355:dbl[])  [unwired: 1 in]
        n248 = Array Max & Min(array=w355) -> (max value=w354:dbl, max index (indices)=w347:i32)  [unwired: 2 out]
        n249 = Greater?(x=w354, y=i8 4) -> (0:w349:bool)
        n250 = case shown="True" w349 {
          tunnel: w347 -> [_ w446]
          tunnel: w352 -> [_ w445]
          tunnel: w348 -> [_ w437]
          tunnel: w346 -> [_ w426]
          tunnel: w345 -> [_ w400]
          tunnel: w344 -> [_ w399]
          tunnel: w343 -> [_ w366]
          tunnel: w342 -> [_ w363]
          tunnel: w341 -> [_ w364]
          tunnel: w340 -> [_ w365]
          frame False {
          }
          frame True {
            n251 = property on="# Events" class="DigNum (strict)"() -> ("Value"=w444:u32)  [unwired: 2 in, 2 out]
            n252 = property on="S1" class="WFGraph (strict)"() -> ("XScale.Offset"=w442:dbl)  [unwired: 2 in, 2 out]
            n253 = property on="S1" class="WFGraph (strict)"() -> ("XScale.Multiplier"=w439:dbl)  [unwired: 2 in, 2 out]
            n254 = Add(x=w445, y=w446) -> (x+y=w415:i32)
            n255 = Add(x=w415, y="WinStart") -> (x+y=w358:i32)
            n256 = Add(x=w415, y="WinEnd") -> (x+y=w423:i32)
            n257 = Index Array(array=w399, index (row)=0) -> (element=w401:dbl[])  [unwired: 1 in]
            n258 = Index Array(array=w366, index (row)=0) -> (element=w389:dbl[])  [unwired: 1 in]
            n259 = Index Array(array=w363, index (row)=0) -> (element=w382:dbl[])  [unwired: 1 in]
            n260 = Index Array(array=w364, index (row)=0) -> (element=w375:dbl[])  [unwired: 1 in]
            n261 = Index Array(array=w365, index (row)=0) -> (element=w368:dbl[])  [unwired: 1 in]
            n262 = Index Array(array=w400, index (row)=0) -> (element=w407:dbl[])  [unwired: 1 in]
            n263 = Index Array(array=w426, index (row)=0) -> (element=w430:dbl[])  [unwired: 1 in]
            n264 = Index Array(array=w437, index (row)=0) -> (element=w414:dbl[])  [unwired: 1 in]
            n265 = Multiply(x=w415, y=w439) -> (x*y=w438:dbl)
            n266 = Increment(x=w444) -> (x+1=w443:u32)
            n267 = Add(x=w442, y=w438) -> (x+y=w413:dbl)
            n268 = Array Subset(array=w407, index=w358, length="WinEnd") -> (w411:dbl[])
            n269 = Array Subset(array=w401, index=w358, length="WinEnd") -> (w405:dbl[])
            n270 = Array Subset(array=w389, index=w358, length="WinEnd") -> (w393:dbl[])
            n271 = Array Subset(array=w382, index=w358, length="WinEnd") -> (w386:dbl[])
            n272 = Array Subset(array=w375, index=w358, length="WinEnd") -> (w379:dbl[])
            n273 = Array Subset(array=w368, index=w358, length="WinEnd") -> (w372:dbl[])
            n274 = Array Subset(array=w430, index=w358, length="WinEnd") -> (w429:dbl[])
            n275 = Array Subset(array=w414, index=w358, length="WinEnd") -> (w435:dbl[])
            n276 = property on="R APB" class="WFGraph (strict)"() -> ("XScale.Multiplier"=w424:dbl)  [unwired: 2 in, 2 out]
            n277 = Array Max & Min(array=w379) -> (max value=w378:dbl, min value=w377:dbl)  [unwired: 2 out]
            n278 = Array Max & Min(array=w372) -> (max value=w371:dbl, min value=w370:dbl)  [unwired: 2 out]
            n279 = Array Max & Min(array=w386) -> (max value=w385:dbl, min value=w384:dbl)  [unwired: 2 out]
            n280 = property on="S1" class="WFGraph (strict)"("Cursor.Cursor X"=w413) -> ()  [unwired: 2 in, 2 out]
            n281 = Array Max & Min(array=w393) -> (max value=w392:dbl, min value=w391:dbl)  [unwired: 2 out]
            n282 = Array Max & Min(array=w411) -> (max value=w410:dbl, min value=w409:dbl)  [unwired: 2 out]
            n283 = Multiply(x=w358, y=w424) -> (x*y=w425:dbl)
            n284 = Array Max & Min(array=w405) -> (max value=w404:dbl, min value=w403:dbl)  [unwired: 2 out]
            n285 = Array Max & Min(array=w429) -> (max value=w428:dbl, min value=w427:dbl)  [unwired: 2 out]
            n286 = Array Max & Min(array=w435) -> (max value=w434:dbl, min value=w433:dbl)  [unwired: 2 out]
            n287 = property on="# Events" class="DigNum (strict)"("Value"=w443) -> ()  [unwired: 2 in, 2 out]
            n288 = Subtract(x=w378, y=w377) -> (x-y=w374:dbl)
            "L BI AMP" <- w374
            n289 = Subtract(x=w371, y=w370) -> (x-y=w367:dbl)
            "L FCR AMP" <- w367
            n290 = Subtract(x=w385, y=w384) -> (x-y=w381:dbl)
            "R FCR AMP" <- w381
            n291 = Subtract(x=w392, y=w391) -> (x-y=w388:dbl)
            "R BI AMP" <- w388
            n292 = Subtract(x=w410, y=w409) -> (x-y=w396:dbl)
            "L APB AMP" <- w396
            n293 = Subtract(x=w404, y=w403) -> (x-y=w395:dbl)
            "L ADM AMP" <- w395
            n294 = Subtract(x=w428, y=w427) -> (x-y=w420:dbl)
            "R ADM AMP" <- w420
            n295 = Subtract(x=w434, y=w433) -> (x-y=w418:dbl)
            "R APB AMP" <- w418
            n296 = property on="AMP Thres" class="DigNum (strict)"() -> ("Value"=w360:dbl)  [unwired: 2 in, 2 out]
            n297 = Multiply(x=w423, y=w424) -> (x*y=w422:dbl)
            n298 = property on="AMP Thres" class="DigNum (strict)"() -> ("Value"=w361:dbl)  [unwired: 2 in, 2 out]
            n299 = property on="AMP Thres" class="DigNum (strict)"() -> ("Value"=w397:dbl)  [unwired: 2 in, 2 out]
            n300 = property on="AMP Thres" class="DigNum (strict)"() -> ("Value"=w362:dbl)  [unwired: 2 in, 2 out]
            n301 = property on="AMP Thres" class="DigNum (strict)"() -> ("Value"=w419:dbl)  [unwired: 2 in, 2 out]
            n302 = property on="AMP Thres" class="DigNum (strict)"() -> ("Value"=w359:dbl)  [unwired: 2 in, 2 out]
            n303 = property on="AMP Thres" class="DigNum (strict)"() -> ("Value"=w398:dbl)  [unwired: 2 in, 2 out]
            n304 = stacked-sequence {
              tunnel: w425 -> [w480 _]
              tunnel: w422 -> [_ w481]
              frame #0 {
                n305 = property on="R APB" class="WFGraph (strict)"("Active Cursor"=u32 0) -> ()  [unwired: 2 in, 2 out]
                n306 = property on="R APB" class="WFGraph (strict)"("Cursor.Cursor X"=w480) -> ()  [unwired: 2 in, 2 out]
              }
              frame #1 {
                n307 = property on="R APB" class="WFGraph (strict)"("Cursor.Cursor X"=w481) -> ()  [unwired: 2 in, 2 out]
                n308 = property on="R APB" class="WFGraph (strict)"("Active Cursor"=u32 1) -> ()  [unwired: 2 in, 2 out]
              }
            }
            n309 = property on="AMP Thres" class="DigNum (strict)"() -> ("Value"=w417:dbl)  [unwired: 2 in, 2 out]
            n310 = Greater Or Equal?(x=w374, y=w360) -> (x >= y?=w376:bool)
            n311 = Greater Or Equal?(x=w367, y=w359) -> (x >= y?=w369:bool)
            n312 = Greater Or Equal?(x=w381, y=w361) -> (x >= y?=w383:bool)
            n313 = Greater Or Equal?(x=w388, y=w362) -> (x >= y?=w390:bool)
            n314 = Greater Or Equal?(x=w396, y=w397) -> (x >= y?=w408:bool)
            n315 = Greater Or Equal?(x=w395, y=w398) -> (x >= y?=w402:bool)
            n316 = Greater Or Equal?(x=w420, y=w419) -> (x >= y?=w416:bool)
            n317 = property on="1st Event Position" class="DigNum (strict)"() -> ("Value"=w441:dbl)  [unwired: 2 in, 2 out]
            n318 = Greater Or Equal?(x=w418, y=w417) -> (x >= y?=w421:bool)
            n319 = case shown="True" w416 {
              frame False {
                n320 = property on="R ADM -" class="DigNum (strict)"() -> ("Value"=w472:i32)  [unwired: 2 in, 2 out]
                n321 = Increment(x=w472) -> (x+1=w471:i32)
                n322 = property on="R ADM -" class="DigNum (strict)"("Value"=w471) -> ()  [unwired: 2 in, 2 out]
              }
              frame True {
                n323 = property on="R ADM +" class="DigNum (strict)"() -> ("Value"=w474:i32)  [unwired: 2 in, 2 out]
                n324 = Increment(x=w474) -> (x+1=w473:i32)
                n325 = property on="R ADM +" class="DigNum (strict)"("Value"=w473) -> ()  [unwired: 2 in, 2 out]
              }
            }
            n326 = case shown="True" w402 {
              frame False {
                n327 = property on="L ADM -" class="DigNum (strict)"() -> ("Value"=w464:i32)  [unwired: 2 in, 2 out]
                n328 = Increment(x=w464) -> (x+1=w463:i32)
                n329 = property on="L ADM -" class="DigNum (strict)"("Value"=w463) -> ()  [unwired: 2 in, 2 out]
              }
              frame True {
                n330 = property on="L ADM +" class="DigNum (strict)"() -> ("Value"=w466:i32)  [unwired: 2 in, 2 out]
                n331 = Increment(x=w466) -> (x+1=w465:i32)
                n332 = property on="L ADM +" class="DigNum (strict)"("Value"=w465) -> ()  [unwired: 2 in, 2 out]
              }
            }
            n333 = case shown="True" w390 {
              frame False {
                n334 = property on="R BI -" class="DigNum (strict)"() -> ("Value"=w460:i32)  [unwired: 2 in, 2 out]
                n335 = Increment(x=w460) -> (x+1=w459:i32)
                n336 = property on="R BI -" class="DigNum (strict)"("Value"=w459) -> ()  [unwired: 2 in, 2 out]
              }
              frame True {
                n337 = property on="R BI +" class="DigNum (strict)"() -> ("Value"=w462:i32)  [unwired: 2 in, 2 out]
                n338 = Increment(x=w462) -> (x+1=w461:i32)
                n339 = property on="R BI +" class="DigNum (strict)"("Value"=w461) -> ()  [unwired: 2 in, 2 out]
              }
            }
            n340 = case shown="True" w408 {
              frame False {
                n341 = property on="L APB -" class="DigNum (strict)"() -> ("Value"=w468:i32)  [unwired: 2 in, 2 out]
                n342 = Increment(x=w468) -> (x+1=w467:i32)
                n343 = property on="L APB -" class="DigNum (strict)"("Value"=w467) -> ()  [unwired: 2 in, 2 out]
              }
              frame True {
                n344 = property on="L APB +" class="DigNum (strict)"() -> ("Value"=w470:i32)  [unwired: 2 in, 2 out]
                n345 = Increment(x=w470) -> (x+1=w469:i32)
                n346 = property on="L APB +" class="DigNum (strict)"("Value"=w469) -> ()  [unwired: 2 in, 2 out]
              }
            }
            n347 = case shown="True" w383 {
              frame False {
                n348 = property on="R FCR -" class="DigNum (strict)"() -> ("Value"=w456:i32)  [unwired: 2 in, 2 out]
                n349 = Increment(x=w456) -> (x+1=w455:i32)
                n350 = property on="R FCR -" class="DigNum (strict)"("Value"=w455) -> ()  [unwired: 2 in, 2 out]
              }
              frame True {
                n351 = property on="R FCR +" class="DigNum (strict)"() -> ("Value"=w458:i32)  [unwired: 2 in, 2 out]
                n352 = Increment(x=w458) -> (x+1=w457:i32)
                n353 = property on="R FCR +" class="DigNum (strict)"("Value"=w457) -> ()  [unwired: 2 in, 2 out]
              }
            }
            n354 = case shown="True" w376 {
              frame False {
                n355 = property on="L BI -" class="DigNum (strict)"() -> ("Value"=w452:i32)  [unwired: 2 in, 2 out]
                n356 = Increment(x=w452) -> (x+1=w451:i32)
                n357 = property on="L BI -" class="DigNum (strict)"("Value"=w451) -> ()  [unwired: 2 in, 2 out]
              }
              frame True {
                n358 = property on="L BI +" class="DigNum (strict)"() -> ("Value"=w454:i32)  [unwired: 2 in, 2 out]
                n359 = Increment(x=w454) -> (x+1=w453:i32)
                n360 = property on="L BI +" class="DigNum (strict)"("Value"=w453) -> ()  [unwired: 2 in, 2 out]
              }
            }
            n361 = case shown="True" w369 {
              frame False {
                n362 = property on="L FCR -" class="DigNum (strict)"() -> ("Value"=w448:i32)  [unwired: 2 in, 2 out]
                n363 = Increment(x=w448) -> (x+1=w447:i32)
                n364 = property on="L FCR -" class="DigNum (strict)"("Value"=w447) -> ()  [unwired: 2 in, 2 out]
              }
              frame True {
                n365 = property on="L FCR +" class="DigNum (strict)"() -> ("Value"=w450:i32)  [unwired: 2 in, 2 out]
                n366 = Increment(x=w450) -> (x+1=w449:i32)
                n367 = property on="L FCR +" class="DigNum (strict)"("Value"=w449) -> ()  [unwired: 2 in, 2 out]
              }
            }
            n368 = Equal To 0?(x=w441) -> (x = 0?=w440:bool)
            n369 = case shown="False" w421 {
              frame False {
                n370 = property on="R APB -" class="DigNum (strict)"() -> ("Value"=w476:i32)  [unwired: 2 in, 2 out]
                n371 = Increment(x=w476) -> (x+1=w475:i32)
                n372 = property on="R APB -" class="DigNum (strict)"("Value"=w475) -> ()  [unwired: 2 in, 2 out]
              }
              frame True {
                n373 = property on="R APB +" class="DigNum (strict)"() -> ("Value"=w478:i32)  [unwired: 2 in, 2 out]
                n374 = Increment(x=w478) -> (x+1=w477:i32)
                n375 = property on="R APB +" class="DigNum (strict)"("Value"=w477) -> ()  [unwired: 2 in, 2 out]
              }
            }
            n376 = case shown="True" w440 {
              tunnel: w413 -> [_ w483]
              frame False {
              }
              frame True {
                n377 = property on="1st Event Position" class="DigNum (strict)"("Value"=w483) -> ()  [unwired: 2 in, 2 out]
              }
            }
          }
        }
      }
    }
    n378 = case shown="1" w251 {
      selector: w251 -> [_ w321 w327 w333 _]
      tunnel: w221 -> [w320 w326 w332 w338 _]
      tunnel: [w320 w326 w332 w338 dbl[][] []] -> w250
      frame 0, Default {
      }
      frame 1 {
        n379 = property on="Rate - every X s" class="DigNum (strict)"() -> ("Value"=w323:dbl)  [unwired: 2 in, 2 out]
        n380 = Multiply(x=36, y=w321) -> (x*y=w324:i32)
        n381 = Multiply(x=w323, y=w324) -> (x*y=w322:dbl)
        n382 = property on="S1" class="WFGraph (strict)"("XScale.Offset"=w322) -> ()  [unwired: 2 in, 2 out]
        n383 = property on="R APB" class="WFGraph (strict)"("XScale.Offset"=w322) -> ()  [unwired: 2 in, 2 out]
        n384 = property on="R ADM" class="WFGraph (strict)"("XScale.Offset"=w322) -> ()  [unwired: 2 in, 2 out]
        n385 = property on="L APB" class="WFGraph (strict)"("XScale.Offset"=w322) -> ()  [unwired: 2 in, 2 out]
        n386 = property on="L ADM" class="WFGraph (strict)"("XScale.Offset"=w322) -> ()  [unwired: 2 in, 2 out]
      }
      frame 2 {
        n387 = property on="Rate - every X s" class="DigNum (strict)"() -> ("Value"=w329:dbl)  [unwired: 2 in, 2 out]
        n388 = Multiply(x=36, y=w327) -> (x*y=w330:i32)
        n389 = Multiply(x=w329, y=w330) -> (x*y=w328:dbl)
        n390 = property on="S1" class="WFGraph (strict)"("XScale.Offset"=w328) -> ()  [unwired: 2 in, 2 out]
        n391 = property on="R APB" class="WFGraph (strict)"("XScale.Offset"=w328) -> ()  [unwired: 2 in, 2 out]
        n392 = property on="R ADM" class="WFGraph (strict)"("XScale.Offset"=w328) -> ()  [unwired: 2 in, 2 out]
        n393 = property on="L APB" class="WFGraph (strict)"("XScale.Offset"=w328) -> ()  [unwired: 2 in, 2 out]
        n394 = property on="L ADM" class="WFGraph (strict)"("XScale.Offset"=w328) -> ()  [unwired: 2 in, 2 out]
      }
      frame 3 {
        n395 = property on="Rate - every X s" class="DigNum (strict)"() -> ("Value"=w335:dbl)  [unwired: 2 in, 2 out]
        n396 = Multiply(x=36, y=w333) -> (x*y=w336:i32)
        n397 = Multiply(x=w335, y=w336) -> (x*y=w334:dbl)
        n398 = property on="S1" class="WFGraph (strict)"("XScale.Offset"=w334) -> ()  [unwired: 2 in, 2 out]
        n399 = property on="R APB" class="WFGraph (strict)"("XScale.Offset"=w334) -> ()  [unwired: 2 in, 2 out]
        n400 = property on="R ADM" class="WFGraph (strict)"("XScale.Offset"=w334) -> ()  [unwired: 2 in, 2 out]
        n401 = property on="L APB" class="WFGraph (strict)"("XScale.Offset"=w334) -> ()  [unwired: 2 in, 2 out]
        n402 = property on="L ADM" class="WFGraph (strict)"("XScale.Offset"=w334) -> ()  [unwired: 2 in, 2 out]
      }
      frame -1 {
      }
    }
    n403 = Compound Arithmetic op=OR(w245, "stop A", "stop B") -> (w244:bool)
    "Samples to Read" <- w307
    "Cursor Auto Jump" <- "Curor Auto Jump"
  }
  n404 = while {
    stop <- w560 stop-if-true
    # "The below part is only for TC trial. It's not a good practice because it takes some parameters from the data aqusition loop."
    # "Button indication"
    # "Change the max to avoid delay greater than buffer size"
    n405 = property class="Bool (strict)"() -> ("Value"=w559:bool)  [unwired: 2 in, 2 out]
    n406 = case shown="True" w559 {
      frame False {
      }
      frame True {
        # "This is to slow down the changing"
        n407 = property on="Looping Iteration" class="DigNum (strict)"() -> ("Value"=w582:i16)  [unwired: 2 in, 2 out]
        n408 = Quotient & Remainder(x=w582, y=i16 4) -> (x-y*floor(x/y)=w579:i16)  [unwired: 1 out]
        n409 = Equal To 0?(x=w579) -> (x = 0?=w580:bool)
        n410 = case shown="True" w580 {
          frame False {
          }
          frame True {
            w588 = FALSE
            n411 = property on="StimulationCounter" class="DigNum (strict)"() -> ("Value"=w584:i32)  [unwired: 2 in, 2 out]
            n412 = property on="Orders" class="Arr (strict)"() -> ("Value"=w601:i32[][])  [unwired: 2 in, 2 out]
            n413 = Array Subset(array=w601, index (row)="?", length (row)=1 ("length")) -> (w598:i32[][])  [unwired: 2 in]
            n414 = Index Array(array=w598, index (row)=0 ("disabled index (row)"), index (col)=w584) -> (element=w587:i32)
            "?" <- w587
            n415 = Decrement(x=w587) -> (x-1=w585:i32)
            n416 = Equal To 0?(x=w585) -> (x = 0?=w586:bool)
            n417 = case shown="False" w586 {
              frame False {
                n418 = property class="RadioBtnsControl (strict)"("Value"=enum32{"ES1", "ES 2", "TMS"}."ES1") -> ()  [unwired: 2 in, 2 out]
              }
              frame True {
                n419 = property class="RadioBtnsControl (strict)"("Value"=enum32{"ES1", "ES 2", "TMS"}."TMS") -> ()  [unwired: 2 in, 2 out]
              }
            }
            n420 = local read "StimulationSetting"() -> (w596:T1)
            n421 = Index Array(array=w596, index=w585) -> (element=w595:T4)
            n422 = Unbundle(w595) -> ("Boolean"=w593:bool, "Boolean"=w592:bool, w591:dbl, w594:dbl, w589:dbl)
            n423 = Add(x=w591, y=w594) -> (x+y=w590:dbl)
            n424 = property on="TMS Activate" class="Bool (strict)"("Value"=w593) -> ()  [unwired: 2 in, 2 out]
            n425 = property on="ES2 Activate" class="Bool (strict)"("Value"=FALSE ("ES2 Activate")) -> ()  [unwired: 2 in, 2 out]
            n426 = property on="ES1 Activate" class="Bool (strict)"("Value"=w592) -> ()  [unwired: 2 in, 2 out]
            n427 = property on="ES1 Delay Interval" class="DigNum (strict)"("Value"=w591) -> ()  [unwired: 2 in, 2 out]
            n428 = property on="TMS Delay Interval" class="DigNum (strict)"("Value"=w589) -> ()  [unwired: 2 in, 2 out]
            n429 = property on="ES2 Delay Interval" class="DigNum (strict)"("Value"=w590) -> ()  [unwired: 2 in, 2 out]
            n430 = property on="ES1 Doublet On?" class="Bool (strict)"("Value"=w588) -> ()  [unwired: 2 in, 2 out]
            n431 = property on="ES2 Doublet On?" class="Bool (strict)"("Value"=w588) -> ()  [unwired: 2 in, 2 out]
            n432 = property on="TMS Doublet On?" class="Bool (strict)"("Value"=w588) -> ()  [unwired: 2 in, 2 out]
          }
        }
      }
    }
    n433 = Divide(x="Buffered Size", y="Sampling Rate") -> (x/y=w574:dbl)
    n434 = case shown="True" "Looping Switch" {
      tunnel: [w604 w614] -> w575
      tunnel: w574 -> [_ w616]
      frame False {
        n435 = local write "Looping Iteration"(0) -> ()
        n436 = case shown="False" "?" {
          tunnel: [1 0] -> w604
          frame False {
          }
          frame True {
          }
        }
      }
      frame True {
        n437 = local read "Looping Iteration"() -> (w618:i16)
        n438 = local read "Repetitions"() -> (w610:i8)
        n439 = Divide(x="Rate - every X s", y=w616) -> (x/y=w619:dbl)
        n440 = Quotient & Remainder(x=w618, y=w619) -> (x-y*floor(x/y)=w614:dbl, floor(x/y)=w613:dbl)
        n441 = Increment(x=w613) -> (x+1=w611:dbl)
        n442 = Equal?(x=w610, y=w611) -> (x = y?=w612:bool)
        n443 = Increment(x=w618) -> (x+1=w617:i16)
        n444 = Subtract(x=w610, y=w611) -> (x-y=→"# Reps Left":dbl)
        n445 = case shown="True" w612 {
          frame False {
          }
          frame True {
            n446 = local write "Looping Switch"(FALSE) -> ()
          }
        }
        n447 = local write "Looping Iteration"(w617) -> ()
      }
    }
    n448 = Multiply(x=w574, y=1000.0) -> (x*y=w564:dbl)
    n449 = property on="ES1 Delay Interval" class="DigNum (strict)"("Maximum"=w564) -> ()  [unwired: 2 in, 2 out]
    n450 = property on="ES 1 Delay Interval (ms)" class="Slide (strict)"("Scale.Maximum"=w564) -> ()  [unwired: 2 in, 2 out]
    n451 = property on="ES2 Delay Interval" class="DigNum (strict)"("Maximum"=w564) -> ()  [unwired: 2 in, 2 out]
    n452 = property on="ES 2 Delay Interval (ms)" class="Slide (strict)"("Scale.Maximum"=w564) -> ()  [unwired: 2 in, 2 out]
    n453 = property on="TMS Delay Interval" class="DigNum (strict)"("Maximum"=w564) -> ()  [unwired: 2 in, 2 out]
    n454 = property on="TMS Delay Interval (ms)" class="Slide (strict)"("Scale.Maximum"=w564) -> ()  [unwired: 2 in, 2 out]
    n455 = Equal To 0?(x=w575) -> (x = 0?=w576:bool)
    n456 = Reciprocal(x="Sampling Rate") -> (1/x=w570:dbl)
    n457 = Multiply(x=w570, y=1000) -> (x*y=w568:dbl)
    n458 = case shown="True" w576 {
      tunnel: [w622 w634] -> w578
      tunnel: "Buffered Size" -> [w621 w635]
      tunnel: w568 -> [_ w632]
      frame False {
        n459 = for {
          N: 3 -> [_]
          tunnel: [w627] -> w622 mode=indexing
          tunnel: w621 -> [w624]
          n460 = Initialize Array(FALSE, w624) -> (w628:bool[])
          n461 = Build Array(w628) -> (w626:bool[][])
          n462 = Transpose 2D Array(2D array=w626) -> (transposed array=w625:bool[][])
          n463 = call-poly <vilib>:"Boolean Array to Digital.vi"("boolean array"=w625) -> ("digital waveform"=w627:digitalwaveform)  [unwired: 9 in, 1 out]
        }
      }
      frame True {
        n464 = for {
          N: 3 -> [_]
          tunnel: [w646] -> w634 mode=indexing
          tunnel: w635 -> [w642]
          tunnel: w632 -> [w641]
          i -> [w643]
          # "Initialize \"off\" for all buffer"
          n465 = Initialize Array(FALSE, w642) -> (w638:bool[])
          n466 = Initialize Array(TRUE, "Trigger Pulse Width (Points)") -> (w639:bool[])
          n467 = case shown="2" w643 {
            tunnel: w641 -> [w653 w682 w711]
            tunnel: w639 -> [w651 w680 w710]
            tunnel: w638 -> [w652 w681 w708]
            tunnel: [w650 w679 w709] -> w637
            tunnel: "Trigger Pulse Width (Points)" -> [w649 w677 w706]
            frame 0, Default {
              n468 = property on="ES1 Activate" class="Bool (strict)"() -> ("Value"=w648:bool)  [unwired: 2 in, 2 out]
              n469 = case shown="True" w648 {
                tunnel: w653 -> [_ w666]
                tunnel: w652 -> [w654 w667]
                tunnel: w651 -> [_ w657]
                tunnel: [w654 w656] -> w650
                tunnel: w649 -> [_ w663]
                frame False {
                }
                frame True {
                  n470 = Divide(x="ES1 Delay Interval", y=w666) -> (x/y=w669:dbl)
                  n471 = property on="ES1 Doublet On?" class="Bool (strict)"() -> ("Value"=w655:bool)  [unwired: 2 in, 2 out]
                  n472 = Round To Nearest(number=w669) -> (nearest integer value=w658:dbl)
                  n473 = Divide(x="ES1 Interval", y=w666) -> (x/y=w664:dbl)
                  n474 = Replace Array Subset(array=w667, new element=w657, index=w658) -> (w660:bool[])
                  n475 = Round To Nearest(number=w664) -> (nearest integer value=w659:dbl)
                  n476 = Greater?(x=w659, y=w663) -> (0:w662:bool)
                  n477 = And(x=w662, y=w655) -> (x .and. y?=w661:bool)
                  n478 = case shown="True" w661 {
                    tunnel: w660 -> [w670 w676]
                    tunnel: w659 -> [_ w674]
                    tunnel: w658 -> [_ w673]
                    tunnel: w657 -> [_ w672]
                    tunnel: [w670 w671] -> w656
                    frame False {
                    }
                    frame True {
                      n479 = Add(x=w673, y=w674) -> (x+y=w675:dbl)
                      n480 = Replace Array Subset(array=w676, new element=w672, index=w675) -> (w671:bool[])
                    }
                  }
                  "ES 1 Delay Interval (ms)" <- "ES1 Delay Interval"
                }
              }
            }
            frame 1 {
              n481 = property on="ES2 Activate" class="Bool (strict)"() -> ("Value"=w678:bool)  [unwired: 2 in, 2 out]
              n482 = case shown="True" w678 {
                tunnel: w681 -> [w683 w697]
                tunnel: w680 -> [_ w686]
                tunnel: [w683 w687] -> w679
                tunnel: w682 -> [_ w689]
                tunnel: w677 -> [_ w690]
                frame False {
                }
                frame True {
                  n483 = Divide(x="ES2 Delay Interval", y=w689) -> (x/y=w698:dbl)
                  n484 = property on="ES2 Doublet On?" class="Bool (strict)"() -> ("Value"=w684:bool)  [unwired: 2 in, 2 out]
                  n485 = Round To Nearest(number=w698) -> (nearest integer value=w685:dbl)
                  n486 = Divide(x="ES2 Interval", y=w689) -> (x/y=w694:dbl)
                  n487 = Replace Array Subset(array=w697, new element=w686, index=w685) -> (w688:bool[])
                  n488 = Round To Nearest(number=w694) -> (nearest integer value=w691:dbl)
                  n489 = Greater?(x=w691, y=w690) -> (0:w693:bool)
                  n490 = And(x=w693, y=w684) -> (x .and. y?=w692:bool)
                  n491 = case shown="True" w692 {
                    tunnel: w688 -> [w699 w705]
                    tunnel: w691 -> [_ w703]
                    tunnel: w685 -> [_ w702]
                    tunnel: w686 -> [_ w701]
                    tunnel: [w699 w700] -> w687
                    frame False {
                    }
                    frame True {
                      n492 = Add(x=w702, y=w703) -> (x+y=w704:dbl)
                      n493 = Replace Array Subset(array=w705, new element=w701, index=w704) -> (w700:bool[])
                    }
                  }
                  "ES 2 Delay Interval (ms)" <- "ES2 Delay Interval"
                }
              }
            }
            frame 2 {
              n494 = property on="TMS Activate" class="Bool (strict)"() -> ("Value"=w707:bool)  [unwired: 2 in, 2 out]
              n495 = case shown="True" w707 {
                tunnel: w708 -> [w712 w726]
                tunnel: w710 -> [_ w717]
                tunnel: [w712 w719] -> w709
                tunnel: w711 -> [_ w715]
                tunnel: w706 -> [_ w716]
                frame False {
                }
                frame True {
                  n496 = Divide(x="TMS Delay Interval", y=w715) -> (x/y=w727:dbl)
                  n497 = property on="TMS Doublet On?" class="Bool (strict)"() -> ("Value"=w713:bool)  [unwired: 2 in, 2 out]
                  n498 = Round To Nearest(number=w727) -> (nearest integer value=w714:dbl)
                  n499 = Divide(x="TMS Interval", y=w715) -> (x/y=w723:dbl)
                  n500 = Replace Array Subset(array=w726, new element=w717, index=w714) -> (w718:bool[])
                  n501 = Round To Nearest(number=w723) -> (nearest integer value=w720:dbl)
                  n502 = Greater?(x=w720, y=w716) -> (0:w722:bool)
                  n503 = And(x=w722, y=w713) -> (x .and. y?=w721:bool)
                  n504 = case shown="True" w721 {
                    tunnel: w718 -> [w728 w734]
                    tunnel: w720 -> [_ w732]
                    tunnel: w714 -> [_ w731]
                    tunnel: w717 -> [_ w730]
                    tunnel: [w728 w729] -> w719
                    frame False {
                    }
                    frame True {
                      n505 = Add(x=w731, y=w732) -> (x+y=w733:dbl)
                      n506 = Replace Array Subset(array=w734, new element=w730, index=w733) -> (w729:bool[])
                    }
                  }
                  "TMS Delay Interval (ms)" <- "TMS Delay Interval"
                }
              }
            }
          }
          n507 = Build Array(w637) -> (w645:bool[][])
          n508 = Transpose 2D Array(2D array=w645) -> (transposed array=w644:bool[][])
          n509 = call-poly <vilib>:"Boolean Array to Digital.vi"("boolean array"=w644) -> ("digital waveform"=w646:digitalwaveform)  [unwired: 9 in, 1 out]
        }
        n510 = property on="StimulationCounter" class="DigNum (strict)"() -> ("Value"=w631:i32)  [unwired: 2 in, 2 out]
        n511 = Increment(x=w631) -> (x+1=w630:i32)
        n512 = property on="StimulationCounter" class="DigNum (strict)"("Value"=w630) -> ()  [unwired: 2 in, 2 out]
      }
    }
    n513 = call "DAQ Assistant"("data"=w578, "rate"="Sampling Rate") -> ()  [unwired: 15 in, 3 out]
    n514 = property on="stop A" class="Bool (strict)"() -> ("Value"=w560:bool)  [unwired: 2 in, 2 out]
    "ES1 On?" <- "ES1 Activate"
    "ES2 On?" <- "ES2 Activate"
    "TMS On?" <- "TMS Activate"
    "ES1 DP On?" <- "ES1 Doublet On?"
    "ES2 DP On?" <- "ES2 Doublet On?"
    "TMS Doublet On?" <- "TMS Doublet On?"
  }
  n515 = Initialize Array(FALSE, 4 ("dimension size")) -> (→"File Writing Array":bool[])
  n516 = property class="Bool (strict)"() -> ("Value"=w22:bool)  [unwired: 2 in, 2 out]
  n517 = case shown="True" w22 {
    tunnel: w13 -> [w736 w739]
    frame False {
      n518 = local read "Single File RefNum"() -> (w737:refnum<file>)
      n519 = Close File(refnum=w737, error in=w736) -> (error out=w735:errorcluster)  [unwired: 1 out]
      n520 = call <vilib>:"Simple Error Handler.vi"("error in (no error)"=w735) -> ()  [unwired: 1 in, 8 out]
    }
    frame True {
      n521 = local read "Files RefNum"() -> (w740:refnum<file>[])
      n522 = property on="Files Opens" class="Arr (strict)"() -> ("Value"=w738:bool[])  [unwired: 2 in, 2 out]
      n523 = for {
        N: 4 -> [_]
        tunnel: w740 -> [w744] mode=indexing
        tunnel: w739 -> [w743]
        tunnel: w738 -> [w742] mode=indexing
        n524 = case shown="True" w742 {
          tunnel: w744 -> [_ w747]
          tunnel: w743 -> [_ w746]
          frame False {
          }
          frame True {
            n525 = Close File(refnum=w747, error in=w746) -> (error out=w745:errorcluster)  [unwired: 1 out]
            n526 = call <vilib>:"Simple Error Handler.vi"("error in (no error)"=w745) -> ()  [unwired: 1 in, 8 out]
          }
        }
      }
    }
  }
  n527 = call <vilib>:"DAQmx Clear Task.vi"("task in"=w47, "error in"=w13) -> ("error out"=w42:errorcluster)  [unwired: 13 out]
  n528 = call <vilib>:"Simple Error Handler.vi"("type of dialog (OK msg:1)"=w43, "error in (no error)"=w42) -> ()  [unwired: 8 out]
  "Looping Iteration" <- w10
  "# Events" <- 0
  "STDP On?" <- "?"
  "1st Event Position" <- u32 0 ("1st Event Position")
  "Group of ES set" <- 0 ("Group of ES set")
  "TC On?" <- "?"
  "StimulationCounter" <- w10
  "R APB +" <- w2
  "R APB -" <- w2
  "R ADM +" <- w2
  "R ADM -" <- w2
  "L APB +" <- w2
  "L APB -" <- w2
  "L ADM +" <- w2
  "L ADM -" <- w2
  "L FCR +" <- w2
  "L FCR -" <- w2
  "L BI -" <- w2
  "L BI +" <- w2
  "R FCR +" <- w2
  "R FCR -" <- w2
  "R BI +" <- w2
  "R BI -" <- w2
